vi "Test1.vi"() -> ()   [LabVIEW 2019]
uses:
  libnewbalancing.dll
panel:
  out "return type":dbl
  in  "Kd":dbl
  in  "Ki":dbl
  in  "Kp":dbl
  in  "rollRate":dbl
  in  "rollRef":dbl
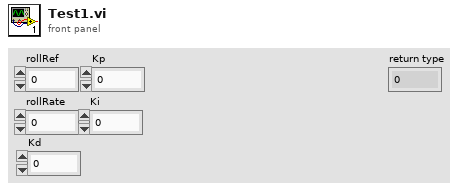
[diagram p1: front panel]
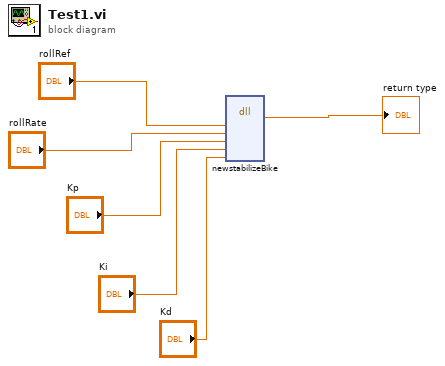
[diagram p0: block diagram]
diagram:
  n1 = dll-call lib="libnewbalancing.*" fn="newstabilizeBike"("rollRef"="rollRef", "rollRate"="rollRate", "Kp"="Kp", "Ki"="Ki", "Kd"="Kd") -> ("return type"=→"return type":dbl)  [unwired: 8 in, 2 out]
